vi "CRYAPI FRAME LIB.vi"(4 "tFrame_In":T2, 6 "tSpliter":T3, 8 "tFrame":T2, 9 "sData":string, 10 "nData":i32, 11 "sAction":string) -> (0 "nData_Out":i32, 1 "sData_Out":string, 2 "tSpliter_Out":T3, 3 "tFrame_Out":T2)   [LabVIEW 2013]
uses:
  <vilib>/Utility/miscctls.llb/LVRectTypeDef.ctl
  CRYMain Sub Window Global.vi
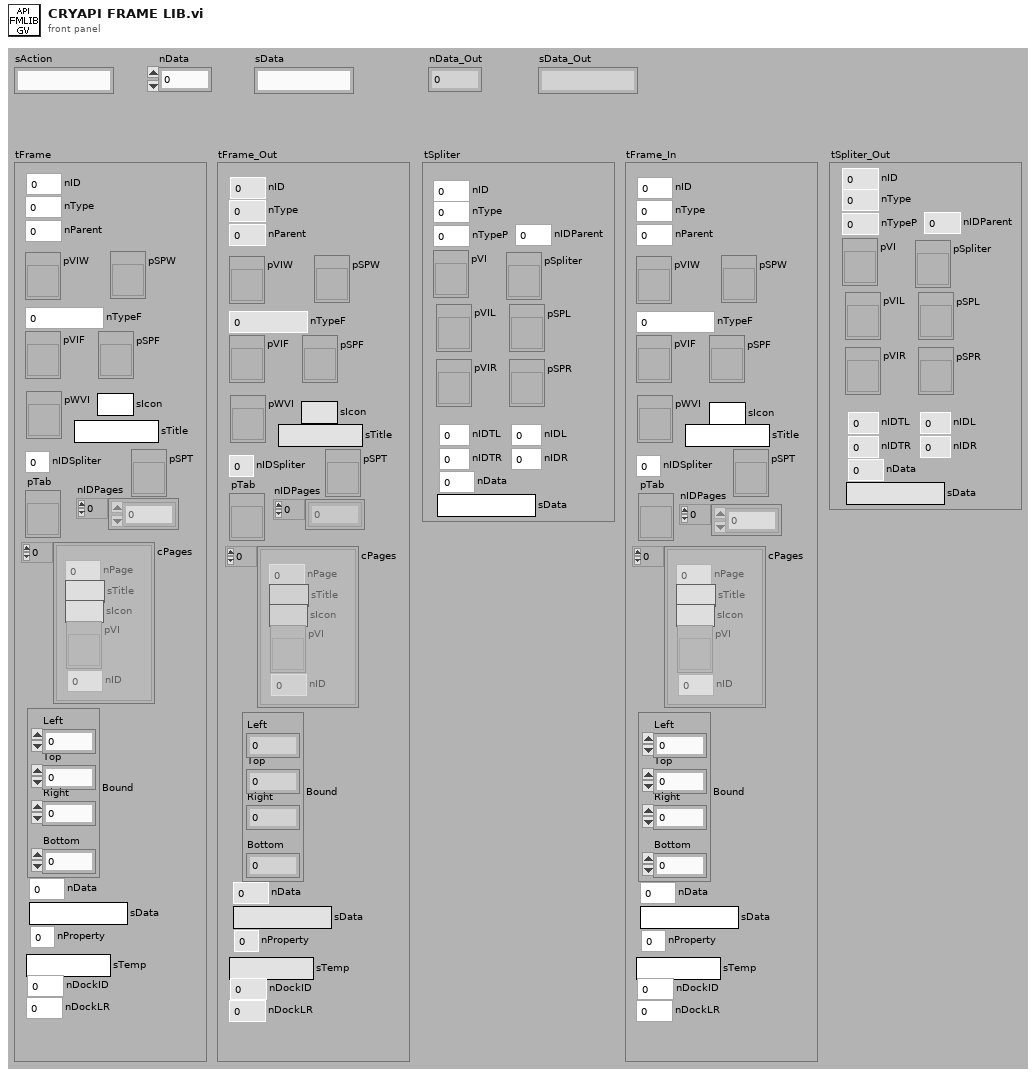
[diagram p1: front panel]
types:
  T1 = typedef "LVRectTypeDef.ctl" = cluster{"Left":i16, "Top":i16, "Right":i16, "Bottom":i16}
  T2 = cluster{"nType":i32, "nParent":i32, "pVIW":refnum<vi>, "pSPW":refnum<vi>, "nTypeF":i32, "pVIF":refnum<vi>, "pSPF":refnum<vi>, "nIDSpliter":i32, "nProperty":i32, "Bound":T1, "nID":i32, "nData":i32, "sData":string, "pWVI":refnum<vi>, "sTitle":string, "cPages":cluster{"nPage":i32, "sTitle":string, "sIcon":string, "pVI":refnum<vi>, "nID":i32}[], "pTab":refnum<vi>, "nIDPages":i32[], "pSPT":refnum<vi>, "sTemp":string, "nDockID":i32, "nDockLR":i32, "sIcon":string}
  T3 = cluster{"nType":i32, "nTypeP":i32, "pVI":refnum<vi>, "pSpliter":refnum<vi>, "pSPL":refnum<vi>, "pVIL":refnum<vi>, "pSPR":refnum<vi>, "pVIR":refnum<vi>, "nIDTL":i32, "nIDL":i32, "nIDTR":i32, "nIDR":i32, "nID":i32, "nIDParent":i32, "nData":i32, "sData":string}
  T4 = cluster{"nPage":i32, "sTitle":string, "sIcon":string, "pVI":refnum<vi>, "nID":i32}[]
  T5 = cluster{"nPage":i32, "sTitle":string, "sIcon":string, "pVI":refnum<vi>, "nID":i32}
  T6 = enum32{"Invalid", "Standard", "Closed", "Hidden", "Minimized", "Maximized"}
  T7 = enum32{"Invalid", "Default", "Floating", "Floating/Auto-Hide", "Modal"}
  T8 = cluster{"CLOSE_HIDE":i32, "CLOSE_CLOSE":i32, "DOCK_ENABLE":i32, "DOCK_DISABLE":i32, "FOCUS_SHOW":i32, "FOCUS_HIDE":i32}
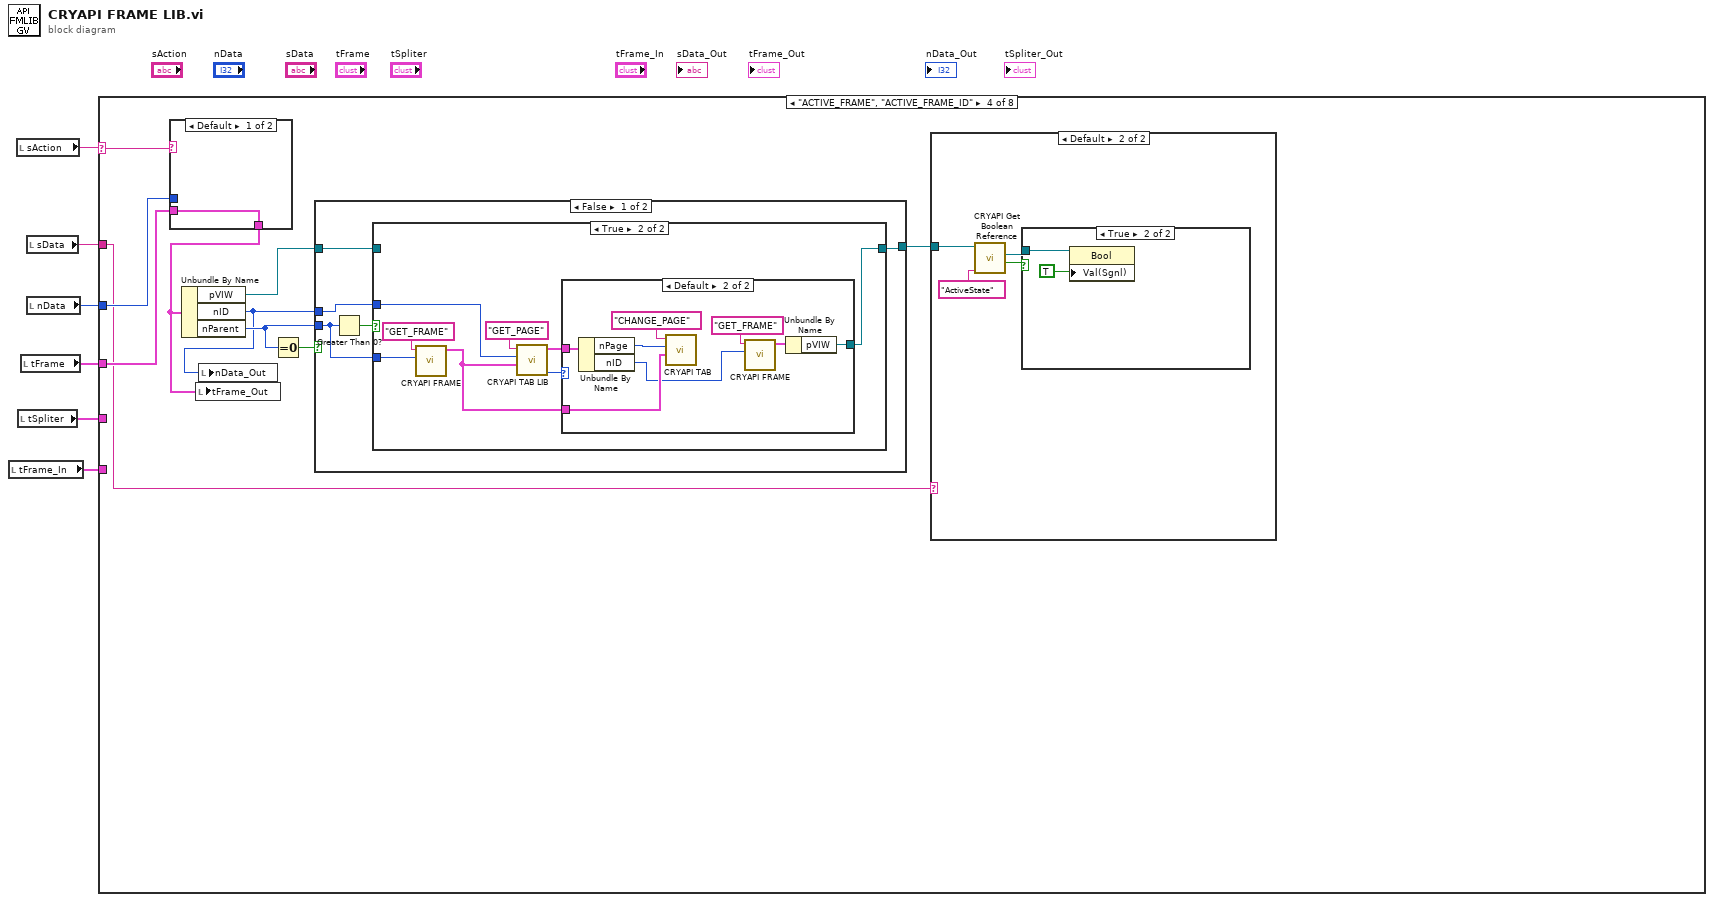
[diagram p0: block diagram]
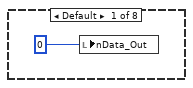
[diagram p2: hidden frame]
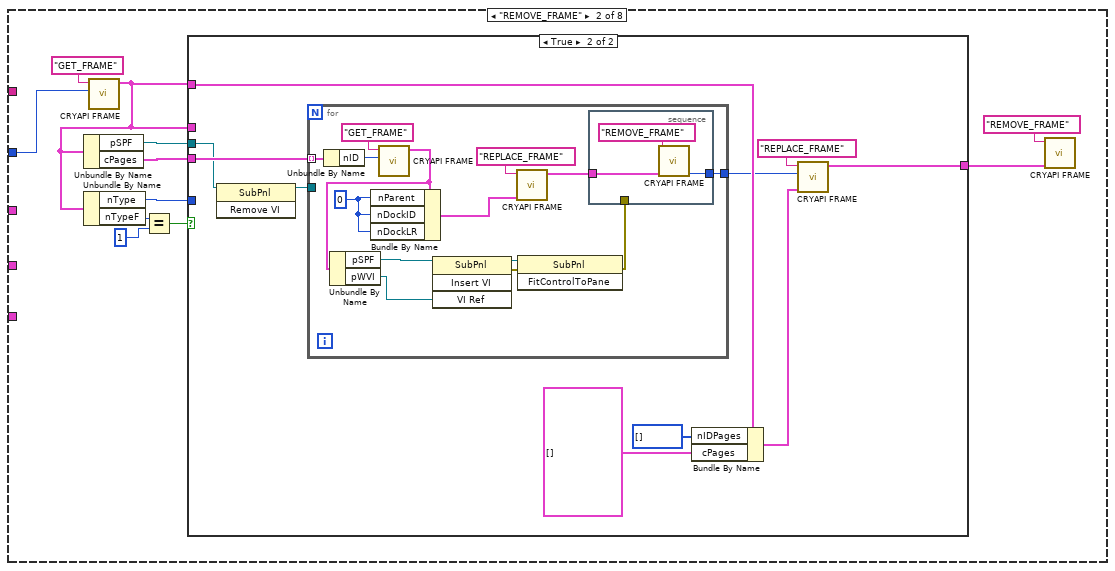
[diagram p3: hidden frame]
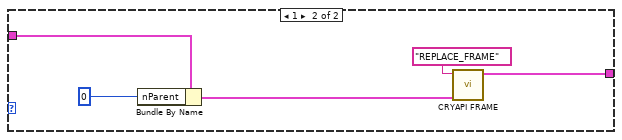
[diagram p5: hidden frame]
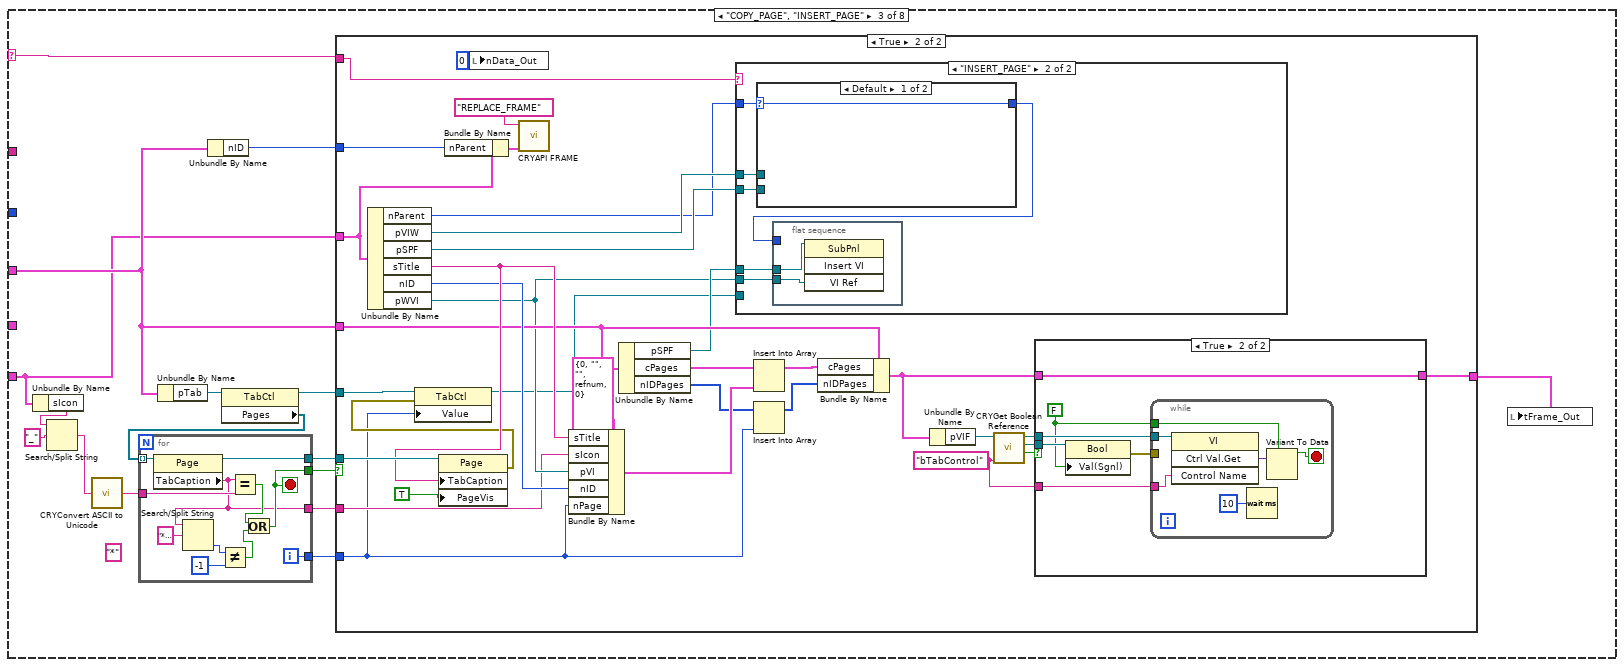
[diagram p6: hidden frame]
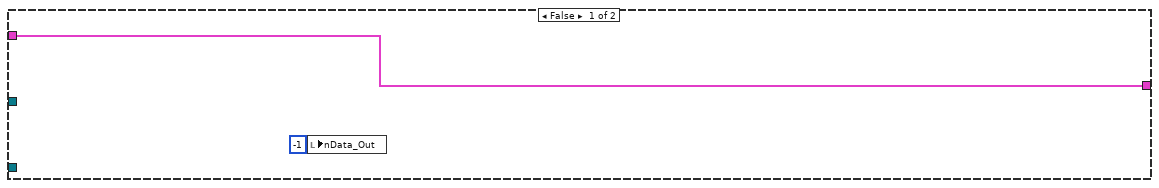
[diagram p7: hidden frame]
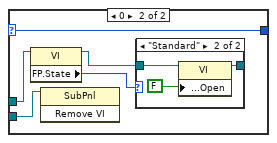
[diagram p10: hidden frame]
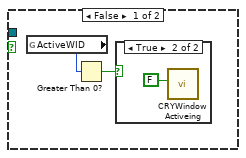
[diagram p13: hidden frame]
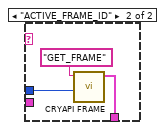
[diagram p15: hidden frame]
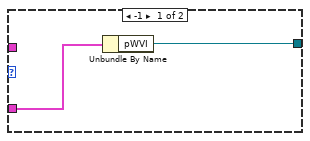
[diagram p17: hidden frame]
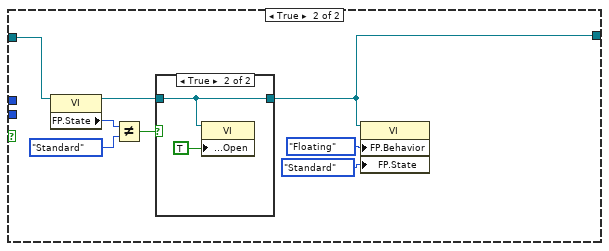
[diagram p18: hidden frame]
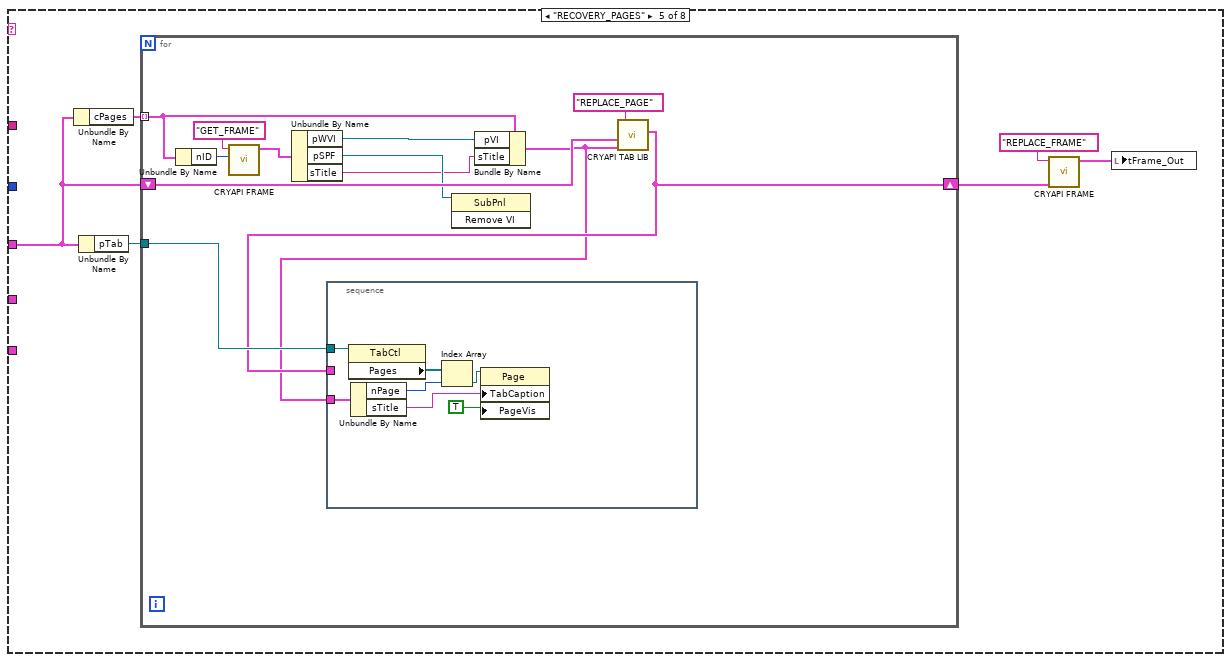
[diagram p20: hidden frame]
diagram:
  n1 = local read "tFrame_In"() -> (w1:T2)
  n2 = local read "sAction"() -> (w6:string)
  n3 = local read "tSpliter"() -> (w2:T3)
  n4 = local read "tFrame"() -> (w3:T2)
  n5 = local read "sData"() -> (w4:string)
  n6 = local read "nData"() -> (w5:i32)
  n7 = case shown="\"ACTIVE_FRAME\", \"ACTIVE_FRAME_ID\"" w6 {
    selector: w6 -> [_ _ w61 w154 _ _ _ _]
    tunnel: w5 -> [_ w12 _ w152 _ _ _ w305]
    tunnel: w4 -> [_ _ _ w151 _ _ _ w293]
    tunnel: w3 -> [_ _ w60 w153 w208 w238 w267 _]
    tunnel: w2 -> [_ _ _ _ _ _ _ _]
    tunnel: w1 -> [_ _ w59 _ _ _ w266 _]
    frame Default {
      n8 = local write "nData_Out"(0 ("nData_Out")) -> ()
    }
    frame "REMOVE_FRAME" {
      n9 = call "CRYAPI FRAME.vi"("nData"=w12, "sAction"="GET_FRAME") -> ("tFrame_Out"=w9:T2)  [unwired: 4 in, 5 out]
      n10 = Unbundle By Name(w9) -> ("pSPF"=w17:refnum<vi>, "cPages"=w16:T4)
      n11 = Unbundle By Name(w9) -> ("nType"=w10:i32, "nTypeF"=w14:i32)
      n12 = Equal?(x=w14, y=1 ("x")) -> (x = y?=w18:bool)
      n13 = case shown="True" w18 {
        tunnel: w9 -> [_ w30]
        tunnel: w16 -> [_ w37]
        tunnel: w17 -> [_ w36]
        tunnel: [w19 w28] -> w11
        tunnel: w10 -> [w21 _]
        tunnel: w9 -> [w20 _]
        frame False {
          n14 = case shown="0, Default" w21 {
            tunnel: w20 -> [w22 w27]
            tunnel: [w22 w24] -> w19
            frame 0, Default {
            }
            frame 1 {
              n15 = Bundle By Name(cluster=w27, "nParent"=0) -> (w23:T2)
              n16 = call "CRYAPI FRAME.vi"("tFrame"=w23, "sAction"="REPLACE_FRAME") -> ("tFrame_Out"=w24:T2)  [unwired: 4 in, 5 out]
            }
          }
        }
        frame True {
          n17 = invoke class="SubPnl" method="Remove VI"(reference=w36) -> (reference out=w35:refnum<vi>)  [unwired: 2 in, 2 out]
          n18 = for {
            tunnel: w37 -> [w51] mode=indexing
            tunnel: w35 -> [_]
            tunnel: [w48] -> w29
            w47 = 0
            n19 = Unbundle By Name(w51) -> ("nID"=w49:i32)
            n20 = call "CRYAPI FRAME.vi"("nData"=w49, "sAction"="GET_FRAME") -> ("tFrame_Out"=w43:T2)  [unwired: 4 in, 5 out]
            n21 = Unbundle By Name(w43) -> ("pSPF"=w42:refnum<vi>, "pWVI"=w41:refnum<vi>)
            n22 = Bundle By Name(cluster=w43, "nParent"=w47, "nDockID"=w47, "nDockLR"=w47) -> (w44:T2)
            n23 = invoke class="SubPnl" method="Insert VI"(reference=w42, "VI Ref"=w41) -> (reference out=w40:refnum<vi>, error out=w39:errorcluster)  [unwired: 2 in, 2 out]
            n24 = call "CRYAPI FRAME.vi"("tFrame"=w44, "sAction"="REPLACE_FRAME") -> ("tFrame_Out"=w45:T2)  [unwired: 4 in, 5 out]
            n25 = invoke class="SubPnl" method="FitControlToPane"(reference=w40, error in=w39) -> (error out=w38:errorcluster)  [unwired: 1 in, 2 out]
            n26 = stacked-sequence {
              tunnel: [w53] -> w48
              tunnel: w45 -> [w52]
              tunnel: w38 -> [_]
              frame #0 {
                n27 = call "CRYAPI FRAME.vi"("tFrame"=w52, "sAction"="REMOVE_FRAME") -> ("nData_Out"=w53:i32)  [unwired: 4 in, 5 out]
              }
            }
          }
          n28 = Bundle By Name(cluster=w30, "nIDPages"=i32[] [], "cPages"=T4 []) -> (w31:T2)
          n29 = call "CRYAPI FRAME.vi"("tFrame"=w31, "nData"=w29, "sAction"="REPLACE_FRAME") -> ("tFrame_Out"=w28:T2)  [unwired: 3 in, 5 out]
        }
      }
      n30 = call "CRYAPI FRAME.vi"("tFrame"=w11, "sAction"="REMOVE_FRAME") -> ()  [unwired: 4 in, 6 out]
    }
    frame "COPY_PAGE", "INSERT_PAGE" {
      (unwired) "*" ("search string/char (-)")
      n31 = Unbundle By Name(w59) -> ("sIcon"=w58:string)
      n32 = Search/Split String(string=w58, search string/char (-)="_") -> (match + rest of string=w57:string)  [unwired: 3 out]
      n33 = call "CRYConvert ASCII to Unicode.vi"("ASCII"=w57) -> ("Unicode"=w56:string)  [unwired: 4 in]
      n34 = Unbundle By Name(w60) -> ("pTab"=w62:refnum<vi>)
      n35 = Unbundle By Name(w60) -> ("nID"=w70:i32)
      n36 = property class="TabCtl"(reference=w62) -> (reference out=w68:refnum<vi>, "Pages"=w67:refnum<vi>[])  [unwired: 1 in, 1 out]
      n37 = for {
        tunnel: w67 -> [w148] mode=indexing
        tunnel: w56 -> [w147]
        tunnel: [w146] -> w64
        tunnel: [w139] -> w63
        tunnel: [w145] -> w65
        tunnel: [w138] -> w69
        i -> [w146]
        stop <- w139 stop-if-true
        n38 = property class="Page"(reference=w148) -> (reference out=w145:refnum<vi>, "TabCaption"=w138:string)  [unwired: 1 in, 1 out]
        n39 = Search/Split String(string=w138, search string/char (-)="*\u0000") -> (offset of match=w143:i32)  [unwired: 3 out]
        n40 = Not Equal?(x=w143, y=-1) -> (x != y?=w140:bool)
        n41 = Equal?(x=w138, y=w147) -> (x = y?=w141:bool)
        n42 = Or(x=w141, y=w140) -> (x .or. y?=w139:bool)
      }
      n43 = case shown="True" w63 {
        tunnel: w60 -> [w71 w95]
        tunnel: [w71 w73] -> w66
        tunnel: w64 -> [_ w80]
        tunnel: w65 -> [_ w104]
        tunnel: w59 -> [_ w86]
        tunnel: w68 -> [_ w96]
        tunnel: w69 -> [_ w88]
        tunnel: w61 -> [_ w87]
        tunnel: w70 -> [_ w85]
        frame False {
          n44 = local write "nData_Out"(-1 ("nData_Out")) -> ()
        }
        frame True {
          w74 = "bTabControl" ("Label Name")
          n45 = Unbundle By Name(w86) -> ("nParent"=w100:i32, "pVIW"=w101:refnum<vi>, "pSPF"=w102:refnum<vi>, "sTitle"=w98:string, "nID"=w97:i32, "pWVI"=w89:refnum<vi>)
          n46 = property class="Page"(reference=w104, "TabCaption"=w98, "PageVis"=TRUE ("Page Visible")) -> (error out=w81:errorcluster)  [unwired: 1 in, 1 out]
          n47 = property class="TabCtl"(reference=w96, error in=w81, "Value"=w80) -> (reference out=w82:refnum<vi>)  [unwired: 1 out]
          n48 = Bundle By Name(cluster=w86, "nParent"=w85) -> (w83:T2)
          n49 = local write "nData_Out"(0 ("nData_Out")) -> ()
          n50 = call "CRYAPI FRAME.vi"("tFrame"=w83, "sAction"="REPLACE_FRAME") -> ()  [unwired: 4 in, 6 out]
          n51 = Bundle By Name(cluster=T5 {"nPage"=0, "sTitle"="", "sIcon"="", "pVI"=refnum, "nID"=0} ("tPage"), "sTitle"=w98, "sIcon"=w88, "pVI"=w89, "nID"=w97, "nPage"=w80) -> (w105:T5)
          n52 = Unbundle By Name(w95) -> ("pSPF"=w90:refnum<vi>, "cPages"=w94:T4, "nIDPages"=w92:i32[])
          n53 = case shown="\"INSERT_PAGE\"" w87 {
            tunnel: w102 -> [_ w125]
            tunnel: w101 -> [_ w124]
            tunnel: w100 -> [_ w123]
            tunnel: w90 -> [_ w122]
            tunnel: w89 -> [_ w121]
            tunnel: w82 -> [_ _]
            frame "COPY_PAGE", Default {
            }
            frame "INSERT_PAGE" {
              n54 = case shown="Default" w123 {
                selector: w123 -> [w128 w129]
                tunnel: w124 -> [_ w131]
                tunnel: w125 -> [_ w130]
                tunnel: [w128 w129] -> w120
                frame Default {
                }
                frame 0 {
                  n55 = property class="VI"(reference=w131) -> (reference out=w133:refnum<vi>, "FP.State"=w132:T6)  [unwired: 1 in, 1 out]
                  n56 = invoke class="SubPnl" method="Remove VI"(reference=w130) -> ()  [unwired: 2 in, 3 out]
                  n57 = case shown="\"Standard\"" w132 {
                    tunnel: w133 -> [w134 w137]
                    tunnel: [w134 w135] -> _
                    frame "Invalid", Default {
                    }
                    frame "Standard" {
                      n58 = property class="VI"(reference=w137, "Front Panel.Open"=FALSE ("Front Panel Window:Open")) -> (reference out=w135:refnum<vi>)  [unwired: 1 in, 1 out]
                    }
                  }
                }
              }
              n59 = flat-sequence {
                tunnel: w122 -> [w127]
                tunnel: w121 -> [w126]
                tunnel: w120 -> [_]
                frame #0 {
                  n60 = invoke class="SubPnl" method="Insert VI"(reference=w127, "VI Ref"=w126) -> ()  [unwired: 2 in, 4 out]
                }
              }
            }
          }
          n61 = Insert Into Array(array=w94, new element=w105) -> (w93:T4)  [unwired: 1 in]
          n62 = Insert Into Array(array=w92, new element=w80) -> (w91:i32[])  [unwired: 1 in]
          n63 = Bundle By Name(cluster=w95, "cPages"=w93, "nIDPages"=w91) -> (w75:T2)
          n64 = Unbundle By Name(w75) -> ("pVIF"=w79:refnum<vi>)
          n65 = call "CRYGet Boolean Reference.vi"("Label Name"=w74, "VI Refnum"=w79) -> ("Exist?"=w78:bool, "Boolean Ref"=w77:refnum<vi>, "VI Refnum Out"=w76:refnum<vi>)  [unwired: 7 in]
          n66 = case shown="True" w78 {
            tunnel: w77 -> [_ w113]
            tunnel: w76 -> [_ w111]
            tunnel: w75 -> [w107 w108]
            tunnel: w74 -> [_ w110]
            tunnel: [w107 w108] -> w73
            frame False {
            }
            frame True {
              w109 = FALSE
              n67 = property class="Bool"(reference=w113, "Val(Sgnl)"=w109) -> (error out=w112:errorcluster)  [unwired: 1 in, 1 out]
              n68 = while {
                tunnel: w112 -> [_]
                tunnel: w111 -> [w119]
                tunnel: w110 -> [w118]
                tunnel: w109 -> [w116]
                stop <- w115 stop-if-true
                n69 = invoke class="VI" method="Ctrl Val.Get"(reference=w119, "Control Name"=w118) -> ("Get Control Value Variant"=w117:variant)  [unwired: 2 in, 3 out]
                n70 = Wait (ms)(milliseconds to wait=u32 10) -> ()  [unwired: 1 out]
                n71 = Variant To Data(type=w116, Variant=w117) -> (data=w115:bool)  [unwired: 1 in, 1 out]
              }
            }
          }
        }
      }
      n72 = local write "tFrame_Out"(w66) -> ()
    }
    frame "ACTIVE_FRAME", "ACTIVE_FRAME_ID" {
      n73 = case shown="Default" w154 {
        tunnel: w153 -> [w168 _]
        tunnel: w152 -> [_ w170]
        tunnel: [w168 w169] -> w150
        frame Default {
        }
        frame "ACTIVE_FRAME_ID" {
          n74 = call "CRYAPI FRAME.vi"("nData"=w170, "sAction"="GET_FRAME") -> ("tFrame_Out"=w169:T2)  [unwired: 4 in, 5 out]
        }
      }
      n75 = Unbundle By Name(w150) -> ("pVIW"=w155:refnum<vi>, "nID"=w149:i32, "nParent"=w158:i32)
      n76 = local write "tFrame_Out"(w150) -> ()
      n77 = local write "nData_Out"(w149) -> ()
      n78 = Equal To 0?(x=w158) -> (x = 0?=w157:bool)
      n79 = case shown="False" w157 {
        tunnel: w155 -> [w174 w203]
        tunnel: [w173 w196] -> w156
        tunnel: w158 -> [w175 _]
        tunnel: w149 -> [w172 _]
        frame False {
          n80 = Greater Than 0?(x=w175) -> (x > 0?=w176:bool)
          n81 = case shown="True" w176 {
            tunnel: w175 -> [_ w184]
            tunnel: w174 -> [w177 _]
            tunnel: [w177 w178] -> w173
            tunnel: w172 -> [_ w182]
            frame False {
            }
            frame True {
              n82 = call "CRYAPI FRAME.vi"("nData"=w184, "sAction"="GET_FRAME") -> ("tFrame_Out"=w179:T2)  [unwired: 4 in, 5 out]
              n83 = call "CRYAPI TAB LIB.vi"("tFrame"=w179, "nData"=w182, "sAction"="GET_PAGE") -> ("nData_Out"=w181:i32, "tPage_Out"=w180:T5)  [unwired: 1 in, 6 out]
              n84 = case shown="Default" w181 {
                tunnel: w180 -> [_ w195]
                tunnel: w179 -> [w187 w192]
                tunnel: [w186 w188] -> w178
                frame -1 {
                  n85 = Unbundle By Name(w187) -> ("pWVI"=w186:refnum<vi>)
                }
                frame Default {
                  n86 = Unbundle By Name(w195) -> ("nPage"=w193:i32, "nID"=w190:i32)
                  n87 = call "CRYAPI TAB.vi"("tFrame"=w192, "nData"=w193, "sAction"="CHANGE_PAGE") -> ()  [unwired: 1 in, 8 out]
                  n88 = call "CRYAPI FRAME.vi"("nData"=w190, "sAction"="GET_FRAME") -> ("tFrame_Out"=w189:T2)  [unwired: 4 in, 5 out]
                  n89 = Unbundle By Name(w189) -> ("pVIW"=w188:refnum<vi>)
                }
              }
            }
          }
        }
        frame True {
          n90 = property class="VI"(reference=w203) -> (reference out=w199:refnum<vi>, "FP.State"=w202:T6)  [unwired: 1 in, 1 out]
          n91 = Not Equal?(x=w202, y=T6."Standard" ("Front Panel Window:State")) -> (x != y?=w200:bool)
          n92 = case shown="True" w200 {
            tunnel: w199 -> [w204 w205]
            tunnel: [w204 w205] -> w196
            frame False {
            }
            frame True {
              n93 = property class="VI"(reference=w205, "Front Panel.Open"=TRUE ("Front Panel Window:Open")) -> ()  [unwired: 1 in, 2 out]
            }
          }
          n94 = property class="VI"(reference=w196, "FP.Behavior"=T7."Floating" ("Front Panel Window:Behavior"), "FP.State"=T6."Standard" ("Front Panel Window:State")) -> ()  [unwired: 1 in, 2 out]
        }
      }
      n95 = case shown="Default" w151 {
        tunnel: w156 -> [_ w162]
        frame "NOFOCUS" {
        }
        frame Default {
          n96 = call "CRYAPI Get Boolean Reference.vi"("Label Name"="ActiveState", "VI Refnum"=w162) -> ("Boolean"=w159:bool, "Boolean Ref"=w161:refnum<vi>)  [unwired: 8 out]
          n97 = case shown="True" w159 {
            tunnel: w161 -> [_ w167]
            frame False {
              n98 = global read "CRYMain Sub Window Global.vi" "ActiveWID"() -> (w164:i32)
              n99 = Greater Than 0?(x=w164) -> (x > 0?=w163:bool)
              n100 = case shown="True" w163 {
                frame False {
                }
                frame True {
                  n101 = call "CRYWindow Activeing.vi"("ActiveTF"=FALSE) -> ()  [unwired: 11 in]
                }
              }
            }
            frame True {
              n102 = property class="Bool"(reference=w167, "Val(Sgnl)"=TRUE) -> ()  [unwired: 1 in, 2 out]
            }
          }
        }
      }
    }
    frame "RECOVERY_PAGES" {
      n103 = Unbundle By Name(w208) -> ("cPages"=w210:T4)
      n104 = Unbundle By Name(w208) -> ("pTab"=w207:refnum<vi>)
      n105 = for {
        tunnel: w210 -> [w217] mode=indexing
        shift-right: [w215] -> w212
        shift-left: w208 -> [w219]
        tunnel: w207 -> [w218]
        n106 = Unbundle By Name(w217) -> ("nID"=w223:i32)
        n107 = call "CRYAPI FRAME.vi"("nData"=w223, "sAction"="GET_FRAME") -> ("tFrame_Out"=w222:T2)  [unwired: 4 in, 5 out]
        n108 = Unbundle By Name(w222) -> ("pWVI"=w221:refnum<vi>, "pSPF"=w216:refnum<vi>, "sTitle"=w214:string)
        n109 = invoke class="SubPnl" method="Remove VI"(reference=w216) -> ()  [unwired: 2 in, 3 out]
        n110 = Bundle By Name(cluster=w217, "pVI"=w221, "sTitle"=w214) -> (w213:T5)
        n111 = call "CRYAPI TAB LIB.vi"("tPage"=w213, "tFrame"=w219, "sAction"="REPLACE_PAGE") -> ("tFrame_Out"=w215:T2)  [unwired: 1 in, 7 out]
        n112 = stacked-sequence {
          tunnel: w218 -> [w227]
          tunnel: w213 -> [w226]
          tunnel: w215 -> [_]
          frame #0 {
            n113 = property class="TabCtl"(reference=w227) -> ("Pages"=w228:refnum<vi>[])  [unwired: 1 in, 2 out]
            n114 = Unbundle By Name(w226) -> ("nPage"=w230:i32, "sTitle"=w225:string)
            n115 = Index Array(array=w228, index=w230) -> (element=w229:refnum<vi>)
            n116 = property class="Page"(reference=w229, "TabCaption"=w225, "PageVis"=TRUE ("Page Visible")) -> ()  [unwired: 1 in, 2 out]
          }
        }
      }
      n117 = call "CRYAPI FRAME.vi"("tFrame"=w212, "sAction"="REPLACE_FRAME") -> ("tFrame_Out"=w209:T2)  [unwired: 4 in, 5 out]
      n118 = local write "tFrame_Out"(w209) -> ()
    }
    frame "REMOVE_SUB---------------" {
      w237 = 1
      n119 = Unbundle By Name(w238) -> ("pWVI"=w245:refnum<vi>)
      n120 = invoke class="VI" method="Ctrl Val.Get"(reference=w245, "Control Name"="SubVI Ref" ("Label Name")) -> ("Get Control Value Variant"=w243:variant)  [unwired: 2 in, 3 out]
      n121 = call "CRYGet Window Subpanel Reference.vi"("Sub Panel Name"="Sub Panel", "VI Ref In"=w245) -> ("SubPnl Refnum"=w247:refnum<vi>)  [unwired: 9 out]
      n122 = invoke class="SubPnl" method="Remove VI"(reference=w247) -> (reference out=w248:refnum<vi>)  [unwired: 2 in, 2 out]
      n123 = Variant To Data(type=w245, Variant=w243) -> (data=w234:refnum<vi>)  [unwired: 1 in, 1 out]
      n124 = call "CRYAPI Get Boolean Reference.vi"("Label Name"="EndFlag", "VI Refnum"=w234) -> ("Boolean"=w233:bool, "Boolean Ref"=w232:refnum<vi>)  [unwired: 8 out]
      n125 = call "CRYAPI Get Boolean Reference.vi"("Label Name"="stop", "VI Refnum"=w234) -> ("Boolean"=w240:bool, "Boolean Ref"=w241:refnum<vi>)  [unwired: 8 out]
      n126 = case shown="True" w240 {
        tunnel: w241 -> [_ w255]
        tunnel: w234 -> [w250 w253]
        tunnel: [w250 w253] -> w244
        tunnel: w248 -> [_ _]
        tunnel: w233 -> [_ w252]
        tunnel: w232 -> [_ w251]
        frame False {
        }
        frame True {
          n127 = To Variant(anything=TRUE) -> (Variant=w254:variant)
          n128 = case shown="True" w252 {
            tunnel: w251 -> [_ w257]
            frame False {
            }
            frame True {
              n129 = while {
                tunnel: w257 -> [w264]
                stop <- w258 stop-if-true
                n130 = property class="Bool"(reference=w264) -> ("Value"=w263:variant)  [unwired: 1 in, 2 out]
                n131 = Variant To Data(type=TRUE, Variant=w263) -> (data=w259:bool, error out=w261:errorcluster)  [unwired: 1 in]
                n132 = Unbundle By Name(w261) -> ("status"=w260:bool)
                n133 = Or(x=w259, y=w260) -> (x .or. y?=w258:bool)
              }
            }
          }
          n134 = property class="Bool"(reference=w255, "Val(Sgnl)"=w254) -> ()  [unwired: 1 in, 2 out]
        }
      }
      n135 = local write "nData_Out"(w237) -> ()
      n136 = Bundle By Name(cluster=w238, "nData"=w237) -> (w249:T2)
      n137 = local write "tFrame_Out"(w249) -> ()
      n138 = call "CRYGet Window Temp Reference.vi"("pVIRef_In"=w244, "sAction"="CLOSE") -> ()  [unwired: 2 in, 8 out]
    }
    frame "RESET_SUB---" {
      n139 = Unbundle By Name(w267) -> ("nData"=w270:i32)
      n140 = Greater Than 0?(x=w270) -> (x > 0?=w269:bool)
      n141 = case shown="True" w269 {
        tunnel: w267 -> [w272 w279]
        tunnel: [w272 w279] -> w268
        tunnel: w267 -> [_ w282]
        tunnel: w266 -> [_ w280]
        tunnel: [0 ("nID") w278] -> w265
        frame False {
        }
        frame True {
          n142 = Unbundle By Name(w280) -> ("pWVI"=w273:refnum<vi>)
          n143 = Unbundle By Name(w282) -> ("pWVI"=w286:refnum<vi>)
          n144 = To Variant(anything=w273) -> (Variant=w284:variant)
          n145 = invoke class="VI" method="Ctrl Val.Set"(reference=w286, "Control Name"="SubVI Ref" ("Label Name"), "Value"=w284) -> ()  [unwired: 2 in, 5 out]
          n146 = call "CRYGet Window Subpanel Reference.vi"("Sub Panel Name"="Sub Panel", "VI Ref In"=w286) -> ("SubPnl Refnum"=w281:refnum<vi>)  [unwired: 9 out]
          n147 = call "CRYGet String Reference.vi"("Label Name"="sVIEWTitle", "VI Refnum"=w273) -> ("Find?"=w276:bool, "VI Refnum Out"=w275:refnum<vi>)  [unwired: 7 in, 1 out]
          n148 = case shown="False" w276 {
            tunnel: w275 -> [w290 w292]
            tunnel: [w289 w292] -> w274
            frame False {
              n149 = invoke class="VI" method="Run VI"(reference=w290, "Wait until done"=FALSE ("Wait Until Done")) -> (reference out=w289:refnum<vi>)  [unwired: 3 in, 4 out]
            }
            frame True {
            }
          }
          n150 = Unbundle By Name(w279) -> ("nID"=w278:i32)
          n151 = invoke class="SubPnl" method="Insert VI"(reference=w281, "VI Ref"=w274) -> (reference out=w287:refnum<vi>, error out=w288:errorcluster)  [unwired: 2 in, 2 out]
          n152 = invoke class="SubPnl" method="FitControlToPane"(reference=w287, error in=w288) -> ()  [unwired: 1 in, 3 out]
        }
      }
      n153 = local write "tFrame_Out"(w268) -> ()
      n154 = local write "nData_Out"(w265) -> ()
    }
    frame "SET_PINSTATE" {
      n155 = global read "CRYMain Sub Window Global.vi" "tWinType"() -> (w295:T8)
      n156 = call "CRYAPI FRAME.vi"("nData"=w305, "sAction"="GET_FRAME") -> ("tFrame_Out"=w296:T2)  [unwired: 4 in, 5 out]
      n157 = Unbundle By Name(w295) -> ("FOCUS_HIDE"=w294:i32)
      n158 = Unbundle By Name(w296) -> ("nID"=w299:i32, "pVIW"=w298:refnum<vi>, "nParent"=w300:i32, "nProperty"=w297:i32)
      n159 = Equal To 0?(x=w300) -> (x = 0?=w302:bool)
      n160 = And(x=w297, y=w294) -> (x .and. y?=w304:i32)
      n161 = Not Equal To 0?(x=w304) -> (x != 0?=w303:bool)
      n162 = And(x=w302, y=w303) -> (x .and. y?=w301:bool)
      n163 = case shown="True" w301 {
        tunnel: w298 -> [_ w308]
        tunnel: w299 -> [_ _]
        tunnel: w293 -> [_ w307]
        frame False {
        }
        frame True {
          n164 = case shown="\"INACTIVE_TRUE\"" w307 {
            tunnel: w308 -> [w312 w321 w330 w339]
            frame "ACTIVE_FALSE", Default {
              n165 = call "CRYAPI Get Boolean Reference.vi"("Label Name"="PinTrue", "VI Refnum"=w312) -> ("Boolean Ref"=w313:refnum<vi>)  [unwired: 9 out]
              n166 = call "CRYAPI Get Boolean Reference.vi"("Label Name"="PinFalse", "VI Refnum"=w312) -> ("Boolean Ref"=w317:refnum<vi>)  [unwired: 9 out]
              n167 = property class="Bool"(reference=w313, "Value"=FALSE ("Visible"), "Visible"=TRUE) -> ()  [unwired: 1 in, 2 out]
              n168 = property class="Bool"(reference=w317, "Value"=FALSE ("Visible"), "Visible"=FALSE) -> ()  [unwired: 1 in, 2 out]
            }
            frame "INACTIVE_FALSE" {
              n169 = call "CRYAPI Get Boolean Reference.vi"("Label Name"="PinTrue", "VI Refnum"=w321) -> ("Boolean Ref"=w322:refnum<vi>)  [unwired: 9 out]
              n170 = call "CRYAPI Get Boolean Reference.vi"("Label Name"="PinFalse", "VI Refnum"=w321) -> ("Boolean Ref"=w326:refnum<vi>)  [unwired: 9 out]
              n171 = property class="Bool"(reference=w322, "Value"=FALSE ("Visible"), "Visible"=FALSE) -> ()  [unwired: 1 in, 2 out]
              n172 = property class="Bool"(reference=w326, "Value"=FALSE ("Visible"), "Visible"=TRUE) -> ()  [unwired: 1 in, 2 out]
            }
            frame "ACTIVE_TRUE" {
              n173 = call "CRYAPI Get Boolean Reference.vi"("Label Name"="PinTrue", "VI Refnum"=w330) -> ("Boolean Ref"=w331:refnum<vi>)  [unwired: 9 out]
              n174 = call "CRYAPI Get Boolean Reference.vi"("Label Name"="PinFalse", "VI Refnum"=w330) -> ("Boolean Ref"=w335:refnum<vi>)  [unwired: 9 out]
              n175 = property class="Bool"(reference=w331, "Value"=TRUE ("Visible"), "Visible"=TRUE) -> ()  [unwired: 1 in, 2 out]
              n176 = property class="Bool"(reference=w335, "Value"=TRUE ("Visible"), "Visible"=FALSE) -> ()  [unwired: 1 in, 2 out]
            }
            frame "INACTIVE_TRUE" {
              n177 = call "CRYAPI Get Boolean Reference.vi"("Label Name"="PinTrue", "VI Refnum"=w339) -> ("Boolean Ref"=w340:refnum<vi>)  [unwired: 9 out]
              n178 = call "CRYAPI Get Boolean Reference.vi"("Label Name"="PinFalse", "VI Refnum"=w339) -> ("Boolean Ref"=w344:refnum<vi>)  [unwired: 9 out]
              n179 = property class="Bool"(reference=w340, "Value"=TRUE ("Visible"), "Visible"=FALSE) -> ()  [unwired: 1 in, 2 out]
              n180 = property class="Bool"(reference=w344, "Value"=TRUE ("Visible"), "Visible"=TRUE) -> ()  [unwired: 1 in, 2 out]
            }
          }
        }
      }
    }
  }
